vi "Init.vi"(7 "Cluster":T1, 8 "error in (no error)":errorcluster, 9 "Init or Array":bool, 10 "Array":dbl[](array[numeric]), 11 "Single Channel in":refnum<class "Single Channel.lvclass">) -> (0 "error out":errorcluster, 3 "Single Channel out":refnum<class "Single Channel.lvclass">)   [LabVIEW 2018, in "Single Channel.lvclass"]
uses:
  Single Channel.lvclass
  Scaling/Scaling.lvclass
  Single Channel.lvclass/Single Channel.ctl
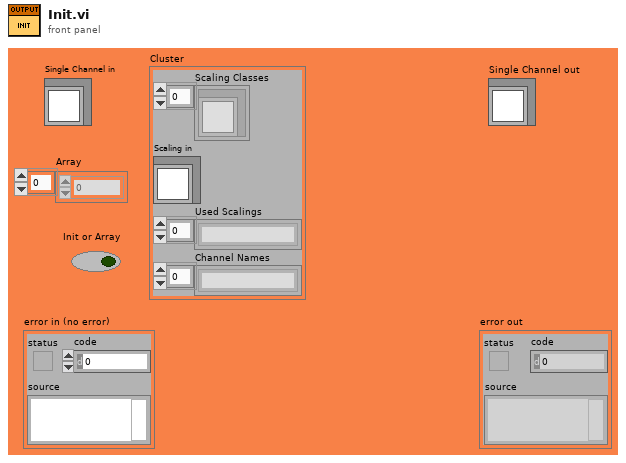
[diagram p1: front panel]
types:
  T1 = cluster{"Scaling Classes":refnum<class "Scaling.lvclass">[], "Scaling in":refnum<class "Scaling.lvclass">, "Used Scalings":string[], "Channel Names":string[]}
  T2 = cluster{"Parsing String":string, "Channel Name":string, "Enabled":bool, "Initial Value":dbl}[]
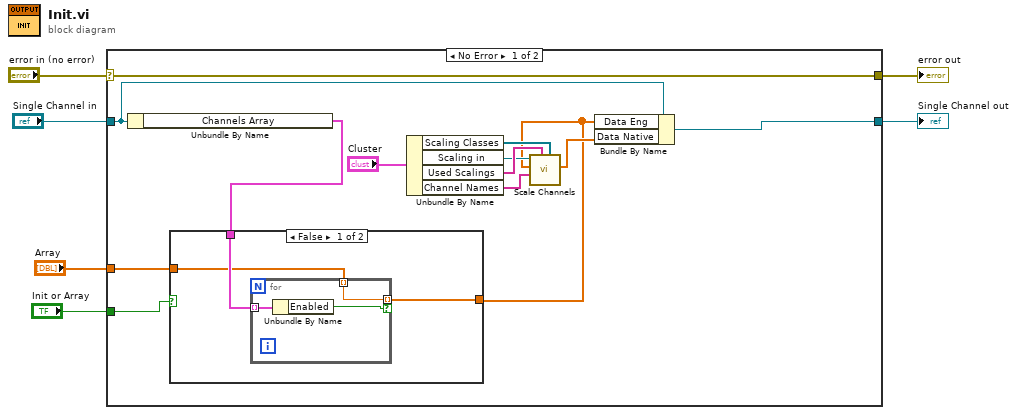
[diagram p0: block diagram]
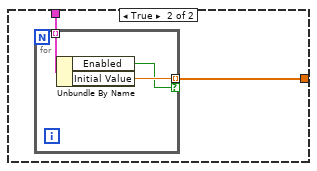
[diagram p2: hidden frame]
diagram:
  n1 = case shown="No Error" "error in (no error)" {
    selector: "error in (no error)" -> [w19 w31]
    tunnel: [w19 w31] -> w5
    tunnel: [w18 w32] -> w4
    tunnel: "Single Channel in" -> [w17 w32]
    tunnel: "Init or Array" -> [w16 _]
    tunnel: "Array" -> [w14 _]
    frame No Error {
      n2 = Unbundle By Name(w17) -> ("Channels Array"=w15:T2)
      n3 = case shown="False" w16 {
        tunnel: w15 -> [w22 w27]
        tunnel: [w21 w26] -> w7
        tunnel: w14 -> [w20 _]
        frame False {
          n4 = for {
            tunnel: w22 -> [w25] mode=indexing
            tunnel: [w24] -> w21 mode=indexing if=w23
            tunnel: w20 -> [w24] mode=indexing
            n5 = Unbundle By Name(w25) -> ("Enabled"=w23:bool)
          }
        }
        frame True {
          n6 = for {
            tunnel: w27 -> [w30] mode=indexing
            tunnel: [w29] -> w26 mode=indexing if=w28
            n7 = Unbundle By Name(w30) -> ("Enabled"=w28:bool, "Initial Value"=w29:dbl)
          }
        }
      }
      n8 = Unbundle By Name("Cluster") -> ("Scaling Classes"=w10:refnum<class "Scaling.lvclass">[], "Scaling in"=w11:refnum<class "Scaling.lvclass">, "Used Scalings"=w12:string[], "Channel Names"=w13:string[])
      n9 = call "Scale Channels.vi"("Scaling Classes"=w10, "Used Scalings"=w12, "Channel Names"=w13, "Values In"=w7, "Scaling in"=w11) -> ("Values Out"=w8:dbl[])  [unwired: 4 in, 2 out]
      n10 = Bundle By Name(cluster=w17, "Data Eng"=w7, "Data Native"=w8) -> (w18:refnum<class "Single Channel.lvclass">)
    }
    frame Error {
    }
  }
  "error out" <- w5
  "Single Channel out" <- w4
